vi "Run Panel VI.vi"(8 "error in (no error)":errorcluster, 11 "Panel in":refnum<class "Panel.lvclass">) -> (0 "error out":errorcluster, 3 "Panel out":refnum<class "Panel.lvclass">)   [LabVIEW 2018, in "OOPanel.lvlib" / "Panel.lvclass"]
uses:
  Panel.lvclass
  Panel.lvclass/Panel.ctl
  State.ctl
  <vilib>/Utility/Data Type/NI_Data Type.lvlib
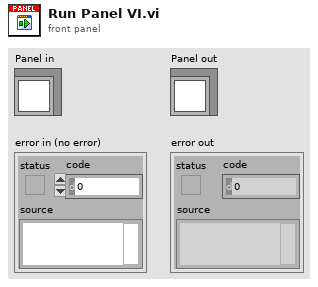
[diagram p1: front panel]
types:
  T1 = typedef "NI_Data Type.lvlib/Data Type.ctl" = enum8{"Invalid Type", "Void", "I8", "I16", "I32", "I64", "U8", "U16", "U32", "U64", "Single Float", "Double Float", "Extended Float", "Single Complex", "Double Complex", "Extended Complex", "Enum U8", "Enum U16", "Enum U32", "Enum U64", "Single Float With Unit", "Double Float With Unit", "Extended Float With Unit", "Single Complex with Unit", "Double Complex with Unit", "Extended Complex with Unit", "Boolean", "String", "Path", "Picture", "Tag", "Array", "Cluster", "Variant", "LV Variant", "Waveform", "Timestamp", "Digital Waveform", "Digital Data", "ExpressData", "Refnum", "External Data", "VI", "Poly VI", "LabVIEW Class Instance", "Fixed Point"}
  T2 = typedef "OOPanel.lvlib/Panel.lvclass/State.ctl" = enum16{"Idle", "Hidden", "Visible", "Subpanel"}
  T3 = typedef "OOPanel.lvlib/Panel.lvclass/Ref Data.ctl" = cluster{"Panel VI":refnum<vi>, "Close":bool, "Panel Events":T4, "Running":bool, "Desired Size":T5, "Subpanel":refnum<vi>, "State":T2}
  T4 = typedef "OOPanel.lvlib/Panel.lvclass/Panel Events.ctl" = cluster{"Close":refnum<user-event>, "Visibility Changed":refnum<user-event>}
  T5 = typedef "OOPanel.lvlib/Panel.lvclass/Desired Size.ctl" = cluster{"Width":i16, "Height":i16}
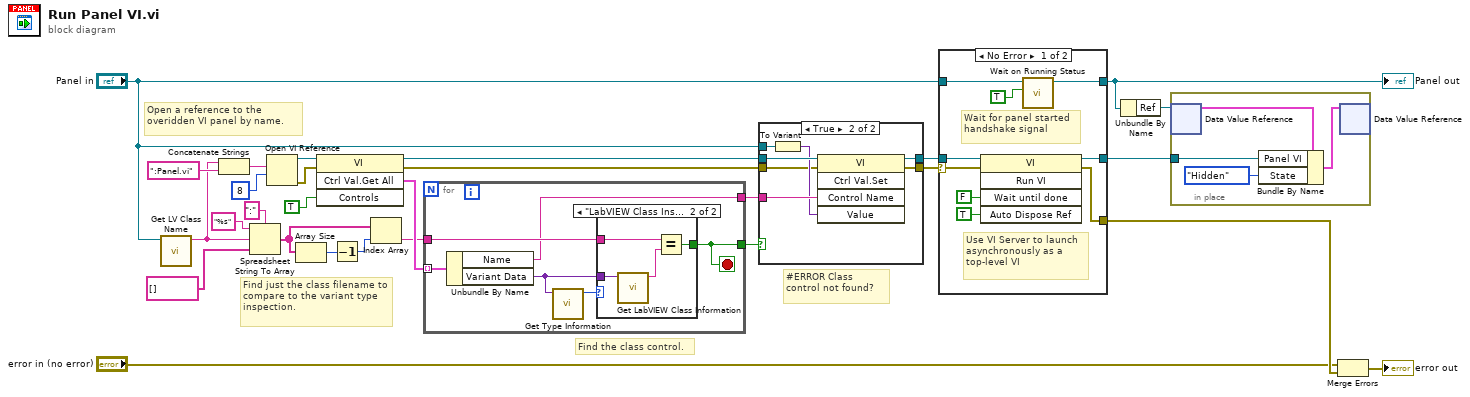
[diagram p0: block diagram]
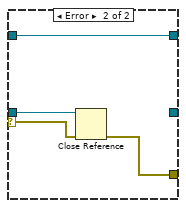
[diagram p2: hidden frame]
diagram:
  # "Find just the class filename to compare to the variant type inspection."
  # "#ERROR Class control not found?"
  # "Find the class control."
  # "Open a reference to the overidden VI panel by name."
  n1 = call <vilib>:"Get LV Class Name.vi"("object"="Panel in") -> ("class name"=w19:string)  [unwired: 9 in, 1 out]
  n2 = Concatenate Strings(w19, ":Panel.vi" ("string")) -> (w23:string)
  n3 = Spreadsheet String To Array(delimiter (Tab)=":", format string="%s", spreadsheet string=w19, array type (2D Dbl)=string[] []) -> (array=w6:string[])
  n4 = Open VI Reference(vi path=w23, options=8) -> (vi reference=w12:refnum<vi>, error out=w22:errorcluster)  [unwired: 4 in]
  n5 = Array Size(array=w6) -> (size(s)=w7:i32)
  n6 = invoke class="VI" method="Ctrl Val.Get All"(reference=w12, error in=w22, "Controls"=TRUE) -> (reference out=w18:refnum<vi>, error out=w15:errorcluster, "Get All Control Values Variant"=w20:cluster{"Name":string, "Variant Data":variant}[])  [unwired: 1 in, 1 out]
  n7 = Decrement(x=w7) -> (x-1=w5:i32)
  n8 = Index Array(array=w6, index=w5) -> (element=w4:string)
  n9 = for {
    tunnel: w20 -> [w34] mode=indexing
    tunnel: w4 -> [w31]
    tunnel: [w30] -> w17
    tunnel: [w29] -> w16
    stop <- w30 stop-if-true
    n10 = Unbundle By Name(w34) -> ("Name"=w29:string, "Variant Data"=w32:variant)
    n11 = call <vilib>:"Get Type Information.vi"("Variant"=w32) -> ("Type"=w33:T1)  [unwired: 6 in, 4 out]
    n12 = case shown="\"LabVIEW Class Instance\"" w33 {
      tunnel: w32 -> [_ w38]
      tunnel: w31 -> [_ w37]
      tunnel: [_ w35] -> w30
      frame Default {
      }
      frame "LabVIEW Class Instance" {
        n13 = call <vilib>:"Get LabVIEW Class Information.vi"("Variant"=w38) -> ("LabVIEW Class File Name"=w36:string)  [unwired: 8 in, 2 out]
        n14 = Equal?(x=w37, y=w36) -> (x = y?=w35:bool)
      }
    }
  }
  n15 = case shown="True" w17 {
    tunnel: w18 -> [w40 w47]
    tunnel: w16 -> [_ w46]
    tunnel: "Panel in" -> [_ w45]
    tunnel: [w39 w43] -> w13
    tunnel: [w40 w42] -> w14
    tunnel: w15 -> [w39 w41]
    frame False {
    }
    frame True {
      n16 = To Variant(anything=w45) -> (Variant=w44:variant)
      n17 = invoke class="VI" method="Ctrl Val.Set"(reference=w47, error in=w41, "Control Name"=w46, "Value"=w44) -> (reference out=w42:refnum<vi>, error out=w43:errorcluster)  [unwired: 1 in, 3 out]
    }
  }
  n18 = case shown="No Error" w13 {
    selector: w13 -> [w53 w59]
    tunnel: w14 -> [w54 w60]
    tunnel: [w51 w58] -> w28
    tunnel: [w52 _] -> w25
    tunnel: "Panel in" -> [w50 w57]
    tunnel: [w49 w57] -> w1
    frame No Error {
      # "Wait for panel started handshake signal"
      # "Use VI Server to launch asynchronously as a top-level VI"
      n19 = invoke class="VI" method="Run VI"(reference=w54, error in=w53, "Wait until done"=FALSE ("Wait Until Done"), "Auto Dispose Ref"=TRUE ("Auto Dispose Reference")) -> (reference out=w52:refnum<vi>, error out=w51:errorcluster)  [unwired: 1 in, 3 out]
      n20 = call "Wait on Running Status.vi"("State"=TRUE, "Panel in"=w50) -> ("Panel out"=w49:refnum<class "Panel.lvclass">)  [unwired: 8 in, 1 out]
    }
    frame Error {
      n21 = Close Reference(reference=w60, error in (no error)=w59) -> (error out=w58:errorcluster)
    }
  }
  "Panel out" <- w1
  n22 = Unbundle By Name(w1) -> ("Ref"=w3:refnum<data-value>)
  n23 = in-place {
    in-place-border: w25 -> [w62]
    n24 = in-place-dvr #1(w3) -> (w64:T3)  [unwired: 1 out]
    n25 = Bundle By Name(cluster=w64, "Panel VI"=w62, "State"=State."Hidden") -> (w63:T3)
    n26 = in-place-dvr #1(w63) -> ()  [unwired: 2 out]
  }
  n27 = Merge Errors("error in (no error)", w28) -> (→"error out":errorcluster)
